vi "Configure IQ Recorder Measurement Trigger.vi"(0 "VISA resource name":refnum<visa-resource-name>, 1 "Timeout (0.5)":dbl=0.5, 2 "Threshold (-30.0)":dbl=-30.0, 5 "Instance (1)":i32=1 format="%.0g", 7 "Source (\"Free Run\")":string="Free Run", 9 "Slope (Rising)":i32(ring) items=["Rising", "Falling"], 11 "error in (no error)":errorcluster, 12 "Offset (0.0001)":dbl=0.0001, 13 "Gap (0.0)":dbl) -> (4 "VISA resource name out":refnum<visa-resource-name>, 15 "error out":errorcluster)   [LabVIEW 2020, in "Rohde&Schwarz CMXP GPRF.lvlib"]
doc: "This VI configures the trigger parameters.\n\nAttributes:\nRSCMXPGPRF_ATTR_IQ_RECORDER_MEASUREMENT_TRIGGER_SOURCE\nRSCMXPGPRF_ATTR_IQ_RECORDER_MEASUREMENT_TRIGGER_SLOPE\nRSCMXPGPRF_ATTR_IQ_RECORDER_MEASUREMENT_TRIGGER_THRESHOLD\nRSCMXPGPRF_ATTR_IQ_RECORDER_MEASUREMENT_TRIGGER_OFFSET\nRSCMXPGPRF_ATTR_IQ_RECORDER_MEASUREMENT_TRIGGER_TIMEOUT\nRSCMXPGPRF_ATTR_IQ_RECORDER_MEASUREMENT_TRIGGER_GAP\n\nRemote-control commands:\nTRIGger:GPRF:MEAS<i>:IQRecorder:SOURce\nTRIGger:GPRF:MEAS<i>:IQRecorder:SLOPe\nTRIGger:GPRF:MEAS<i>:IQRecorder:THReshold\nTRIGger:GPRF:MEAS<i>:IQRecorder:OFFSet\nTRIGger:GPRF:MEAS<i>:IQRecorder:TOUT\nTRIGger:GPRF:MEAS<i>:IQRecorder:MGAP"
uses:
  <instrlib>/Rohde&Schwarz CMXP GPRF/Rohde&Schwarz CMXP GPRF.lvlib
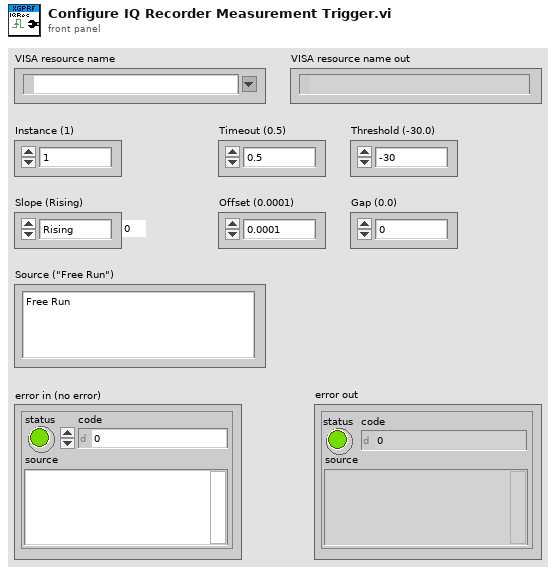
[diagram p1: front panel]
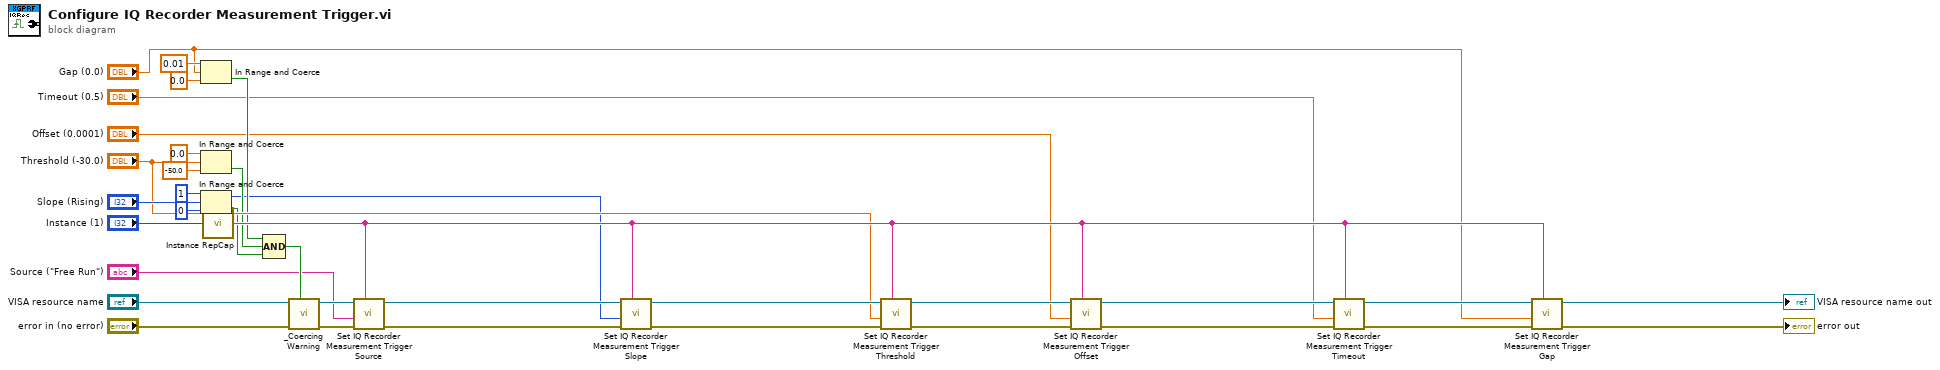
[diagram p0: block diagram]
diagram:
  n1 = In Range and Coerce(upper limit=0.01, x="Gap (0.0)", lower limit=0.0) -> (In Range?=w5:bool)  [unwired: 1 out]
  n2 = In Range and Coerce(upper limit=0.0, x="Threshold (-30.0)", lower limit=-50.0) -> (In Range?=w6:bool)  [unwired: 1 out]
  n3 = In Range and Coerce(upper limit=1, x="Slope (Rising)", lower limit=0) -> (coerced(x)=w2:i32, In Range?=w7:bool)
  n4 = call <instrlib>:"Instance RepCap.vi"("Instance in"="Instance (1)") -> ("Instance out"=w10:string)
  n5 = Compound Arithmetic op=AND(w5, w6, w7) -> (w25:bool)
  n6 = call <instrlib>:"_Coercing Warning.vi"("In Range?"=w25, "error in (no error)"="error in (no error)", "VISA resource name"="VISA resource name") -> ("error out"=w23:errorcluster, "VISA resource name out"=w24:refnum<visa-resource-name>)  [unwired: 7 in]
  n7 = call "Set IQ Recorder Measurement Trigger Source"("Repeated Capabilities"=w10, "error in (no error)"=w23, "IQ Recorder Measurement Trigger Source ()"="Source (\"Free Run\")", "instrument handle"=w24) -> ("error out"=w21:errorcluster, "instrument handle out"=w22:refnum<visa-resource-name>)  [unwired: 6 in]
  n8 = call "Set IQ Recorder Measurement Trigger Slope"("Repeated Capabilities"=w10, "error in (no error)"=w21, "IQ Recorder Measurement Trigger Slope (0 - Rising)"=w2, "instrument handle"=w22) -> ("error out"=w19:errorcluster, "instrument handle out"=w20:refnum<visa-resource-name>)  [unwired: 6 in]
  n9 = call "Set IQ Recorder Measurement Trigger Threshold"("Repeated Capabilities"=w10, "error in (no error)"=w19, "IQ Recorder Measurement Trigger Threshold (0.0)"="Threshold (-30.0)", "instrument handle"=w20) -> ("error out"=w17:errorcluster, "instrument handle out"=w18:refnum<visa-resource-name>)  [unwired: 6 in]
  n10 = call "Set IQ Recorder Measurement Trigger Offset"("Repeated Capabilities"=w10, "error in (no error)"=w17, "IQ Recorder Measurement Trigger Offset (0.0)"="Offset (0.0001)", "instrument handle"=w18) -> ("error out"=w15:errorcluster, "instrument handle out"=w16:refnum<visa-resource-name>)  [unwired: 6 in]
  n11 = call "Set IQ Recorder Measurement Trigger Timeout"("Repeated Capabilities"=w10, "error in (no error)"=w15, "IQ Recorder Measurement Trigger Timeout (0.0)"="Timeout (0.5)", "instrument handle"=w16) -> ("error out"=w13:errorcluster, "instrument handle out"=w14:refnum<visa-resource-name>)  [unwired: 6 in]
  n12 = call "Set IQ Recorder Measurement Trigger Gap"("Repeated Capabilities"=w10, "error in (no error)"=w13, "IQ Recorder Measurement Trigger Gap (0.0)"="Gap (0.0)", "instrument handle"=w14) -> ("error out"=→"error out":errorcluster, "instrument handle out"=→"VISA resource name out":refnum<visa-resource-name>)  [unwired: 6 in]
